vi "DB connected in local host.vi"(8 "error in (no error)":errorcluster, 11 "Refnum in":T1) -> (0 "error out":errorcluster, 3 "DB Connected":bool)   [LabVIEW 2024, in "DB.lvlib"]
uses:
  DB.lvlib
  <vilib>/addons/database/Connection.llb/Conn ObjectReference.ctl
  <vilib>/addons/database/Connection.llb/Conn Execute.vi
  <vilib>/addons/database/Recordset.llb/Rec Fetch Recordset Data (R).vi
  <userlib>/_OpenG.lib/array/array.llb/Search 1D Array (Boolean)__ogtk.vi
  <vilib>/addons/database/NI_Database_API.lvlib
  <userlib>/_OpenG.lib/array/array.llb/openg_array.lvlib
panel:
  out "size(s) 2":i32
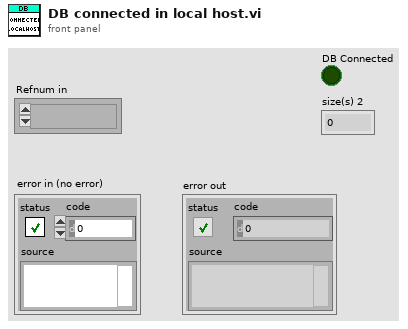
[diagram p1: front panel]
types:
  T1 = typedef "NI_Database_API.lvlib/Conn ObjectReference.ctl" = refnum<k1>
  T2 = typedef "NI_Database_API.lvlib/Rec ObjectReference.ctl" = refnum<k1>
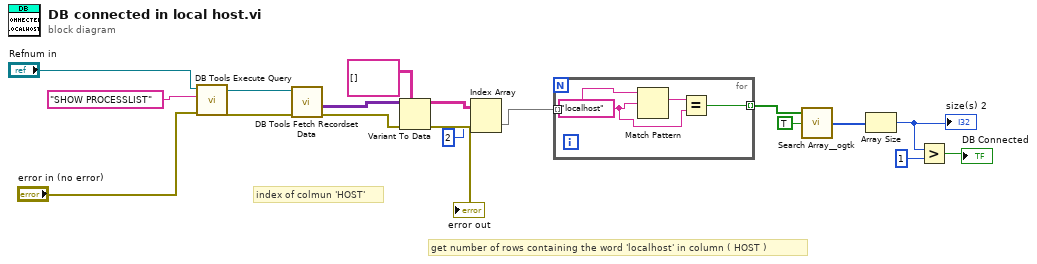
[diagram p0: block diagram]
diagram:
  # "index of colmun 'HOST'"
  # "get number of rows containing the word 'localhost' in column ( HOST )"
  n1 = call-poly <vilib>:"DB Tools Execute Query.vi"("error in (no error)"="error in (no error)", "SQL query"="SHOW PROCESSLIST", "connection reference"="Refnum in") -> ("error out"=w11:errorcluster, "recordset reference"=w10:T2)  [unwired: 5 in]
  n2 = call-poly <vilib>:"DB Tools Fetch Recordset Data.vi"("error in (no error)"=w11, "recordset reference"=w10) -> ("error out"=w16:errorcluster, "recordset data"=w12:variant[][])  [unwired: 3 in, 1 out]
  n3 = Variant To Data(error in=w16, type=string[][] [], Variant=w12) -> (data=w14:string[][], error out=→"error out":errorcluster)
  n4 = Index Array(array=w14, index (col)=2 ("disabled index (col)")) -> (element=w5:string[])  [unwired: 1 in]
  n5 = for {
    tunnel: w5 -> [w22] mode=indexing
    tunnel: [w19] -> w7 mode=indexing
    w20 = "localhost" ("regular expression")
    n6 = Match Pattern(string=w22, regular expression=w20) -> (match substring=w21:string)  [unwired: 1 in, 3 out]
    n7 = Equal?(x=w21, y=w20) -> (x = y?=w19:bool)
  }
  n8 = call-poly <userlib>:"Search Array__ogtk.vi"("Array"=w7, "Element Data"=TRUE) -> ("Indices of Elements"=w4:i32[])  [unwired: 7 in]
  n9 = Array Size(array=w4) -> (size(s)=w3:i32)
  "size(s) 2" <- w3
  n10 = Greater?(x=w3, y=1) -> (0:→"DB Connected":bool)
